vi "Experiment header-Bundle & save STATS section.vi"(8 "error in (no error)":errorcluster, 11 "Logging queue element":T1 {"Ref Dwell time (us)" format="%#.6g"; "Frame Size" items=["100X100"=100, "128X128"=128, "200X200"=200, "256X256"=256, "512X512"=512, "1024x1024"=1024, "2048x2048"=2048]; "Dwell time (us)" format="%#.6g"}) -> (0 "error out":errorcluster)   [LabVIEW 2017]
uses:
  Typedefs/Logging queue element.ctl
  Typedefs/Imaging Protocols enum.ctl
  Typedefs/Frame Size.ctl
  Typedefs/Acquired points count.ctl
  Global Variables/General Globals.vi
panel:
  in  "Array":u64[](array[numeric])
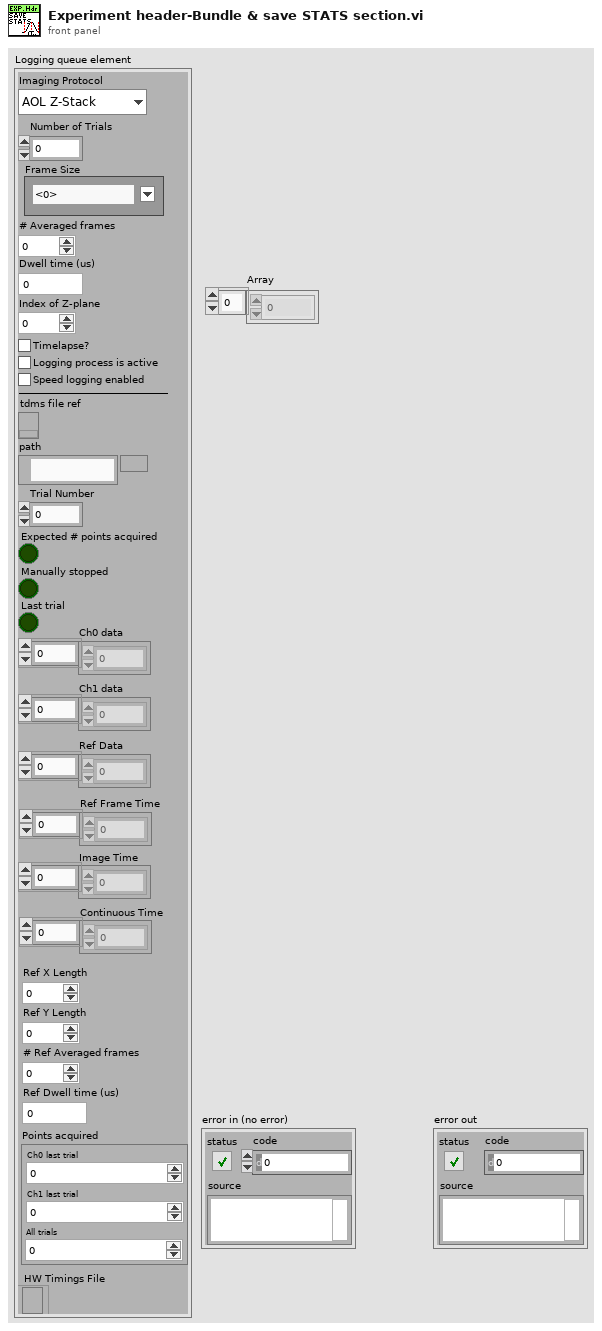
[diagram p1: front panel]
types:
  T1 = typedef "Logging queue element.ctl" = cluster{"Imaging Protocol":T2, "Number of Trials":u16, "Frame Size":T3, "# Averaged frames":u16, "Dwell time (us)":dbl, "Index of Z-plane":i32, "Timelapse?":bool, "Logging process is active":bool, "Speed logging enabled":bool, "tdms file ref":refnum<k34>, "path":path, "Trial Number":i32, "Expected # points acquired":bool, "Manually stopped":bool, "Last trial":bool, "Ch0 data":u32[], "Ch1 data":u32[], "Ref Data":u32[], "Ref Frame Time":u64[], "Image Time":u64[], "Continuous Time":u64[], "Ref X Length":u16, "Ref Y Length":u16, "# Ref Averaged frames":u16, "Ref Dwell time (us)":dbl, "Points acquired":T4, "HW Timings File":refnum<file>}
  T2 = typedef "Imaging Protocols enum.ctl" = enum16{"AOL Z-Stack", "Motor Z Stack", "Functional Acquisition", "Single Plane Acquisition", "Volume Acquisition", "Live Imaging", "Live Plane Imaging", "Live Volume Imaging"}
  T3 = typedef "Frame Size.ctl" = u16
  T4 = typedef "Acquired points count.ctl" = cluster{"Ch0 last trial":u64, "Ch1 last trial":u64, "All trials":u64}
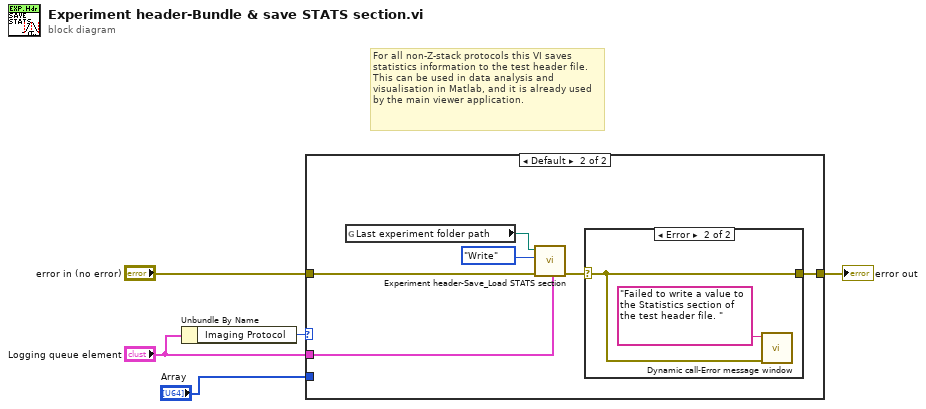
[diagram p0: block diagram]
diagram:
  # "For all non-Z-stack protocols this VI saves statistics information to the test header file.\nThis can be used in data analysis and visualisation in Matlab, and it is already used by the main viewer application."
  n1 = Unbundle By Name("Logging queue element") -> ("Imaging Protocol"=w3:T2)
  n2 = case shown="Default" w3 {
    tunnel: [w6 w7] -> w5
    tunnel: "error in (no error)" -> [w6 w12]
    tunnel: "Logging queue element" -> [_ w11]
    tunnel: "Array" -> [_ _]
    frame "AOL Z-Stack", "Motor Z Stack" {
    }
    frame Default {
      n3 = global read "General Globals.vi" "Last experiment folder path"() -> (w9:path)
      n4 = call "Experiment header-Save_Load STATS section.vi"("Logging queue element"=w11, "error in (no error)"=w12, "Function"=enum16{"Write", "Read"}."Write", "Experiment folder path"=w9) -> ("error out"=w8:errorcluster)  [unwired: 5 in, 2 out]
      n5 = case shown="Error" w8 {
        selector: w8 -> [w13 w14]
        tunnel: [w13 w14] -> w7
        frame No Error {
        }
        frame Error {
          n6 = call "Dynamic call-Error message window.vi"("error in (no error)"=w14, "Error Message"="Failed to write a value to the Statistics section of the test header file. ") -> ()  [unwired: 9 in, 1 out]
        }
      }
    }
  }
  "error out" <- w5
